vi "DataVIS_Update_Cursor.vi"(8 "error in (no error)":errorcluster, 9 "Cursor Graph":refnum<vi>, 10 "Field / temp":i32, 11 "Visualize Data Cluster IN":T2) -> (0 "error out":errorcluster, 1 "Field":dbl=-3.687258687258687, 2 "slowest":dbl=4.2894631624221803e-07, 3 "Visualize Data Cluster OUT":T2)   [LabVIEW 2016]
uses:
  <vilib>/Utility/miscctls.llb/LVPointDoubleTypeDef.ctl
panel:
  in  "Field/Temperature 2":refnum<vi>
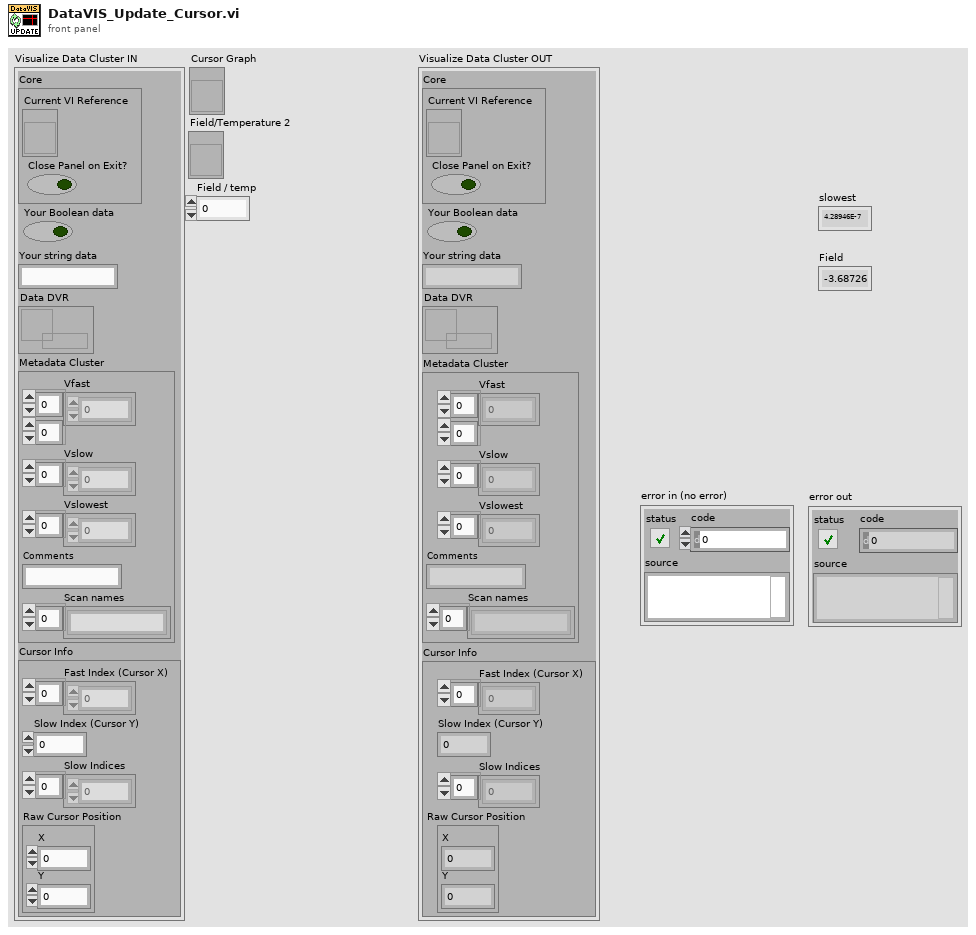
[diagram p1: front panel]
types:
  T1 = typedef "LVPointDoubleTypeDef.ctl" = cluster{"X":dbl, "Y":dbl}
  T2 = cluster{"Core":cluster{"Current VI Reference":refnum<vi>, "Close Panel on Exit?":bool}, "Your Boolean data":bool, "Your string data":string, "Data DVR":refnum<data-value>, "Metadata Cluster":cluster{"Vfast":dbl[][], "Vslow":dbl[], "Vslowest":dbl[], "Comments":string, "Scan names":string[]}, "Cursor Info":cluster{"Fast Index (Cursor X)":dbl[], "Slow Index (Cursor Y)":dbl, "Slow Indices":dbl[], "Raw Cursor Position":T1}}
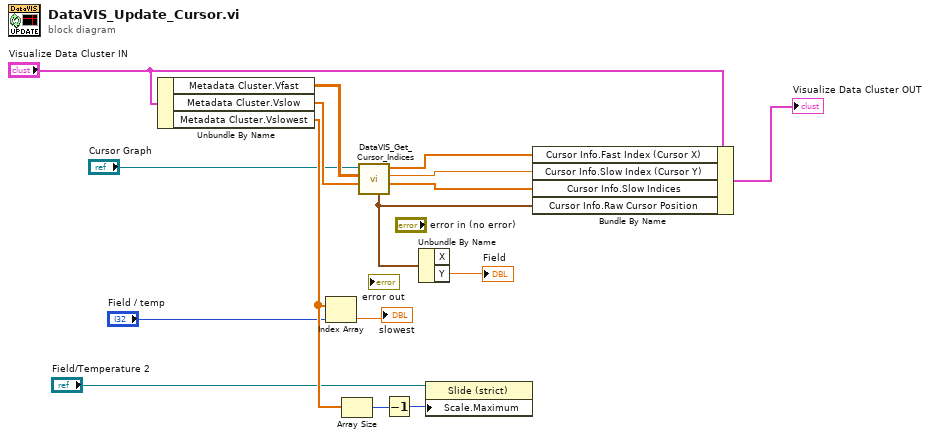
[diagram p0: block diagram]
diagram:
  n1 = Unbundle By Name("Visualize Data Cluster IN") -> ("Metadata Cluster.Vfast"=w16:dbl[][], "Metadata Cluster.Vslow"=w15:dbl[], "Metadata Cluster.Vslowest"=w10:dbl[])
  n2 = Index Array(array=w10, index="Field / temp") -> (element=→"slowest":dbl)
  n3 = Array Size(array=w10) -> (size(s)=w14:i32)
  n4 = call "DataVIS_Get_Cursor_Indices.vi"("Vslow"=w15, "Vfast"=w16, "Cursor Graph"="Cursor Graph") -> ("Slow Indices"=w7:dbl[], "Slow Index (Cursor Y)"=w8:dbl, "Fast Index (Cursor X) (IDK why it's an array)"=w9:dbl[], "Raw Cursor Position"=w6:T1)  [unwired: 4 in, 1 out]
  n5 = Decrement(x=w14) -> (x-1=w13:i32)
  n6 = Unbundle By Name(w6) -> ("Y"=→"Field":dbl)  [unwired: 1 out]
  n7 = property on="Property Node" class="Slide (strict)"(reference="Field/Temperature 2", "Scale.Maximum"=w13) -> ()  [unwired: 1 in, 2 out]
  n8 = Bundle By Name(cluster="Visualize Data Cluster IN", "Cursor Info.Fast Index (Cursor X)"=w9, "Cursor Info.Slow Index (Cursor Y)"=w8, "Cursor Info.Slow Indices"=w7, "Cursor Info.Raw Cursor Position"=w6) -> (→"Visualize Data Cluster OUT":T2)
